vi "Sort-Number.vi"() -> ()   [LabVIEW 2014]
panel:
  out "sorted array\n(From large to small)":dbl[](array[numeric])
  out "sorted array\n(From small to large )":dbl[](array[numeric])
  in  "Input number":dbl[](array[numeric])
  in  "stop":bool
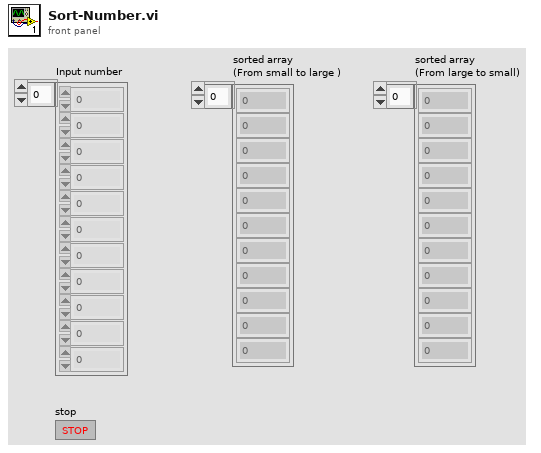
[diagram p1: front panel]
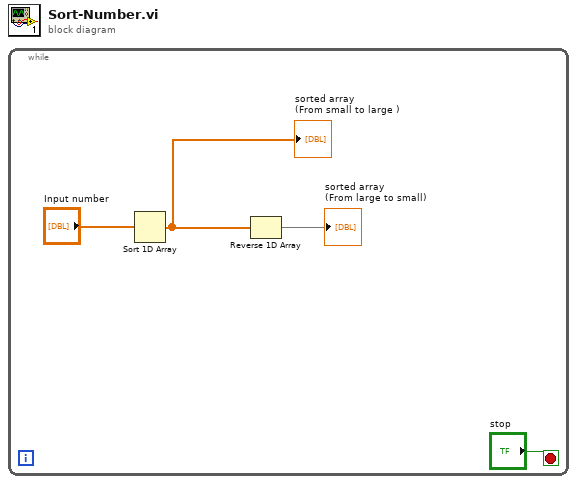
[diagram p0: block diagram]
diagram:
  n1 = while {
    stop <- "stop" stop-if-true
    n2 = Sort 1D Array(array="Input number") -> (sorted array=w1:dbl[])
    "sorted array\n(From small to large )" <- w1
    n3 = Reverse 1D Array(array=w1) -> (reversed array=→"sorted array\n(From large to small)":dbl[])
  }
